vi "get desired keys.vi"(8 "error in":errorcluster, 11 "MotionModule configuration in":refnum<class "MotionModule configuration.lvclass">) -> (0 "error out":errorcluster, 2 "desired keys":string[](array[string]), 3 "MotionModule configuration out":refnum<class "MotionModule configuration.lvclass">)   [LabVIEW 2017, in "MotionModule configuration.lvclass"]
uses:
  MotionModule configuration.lvclass
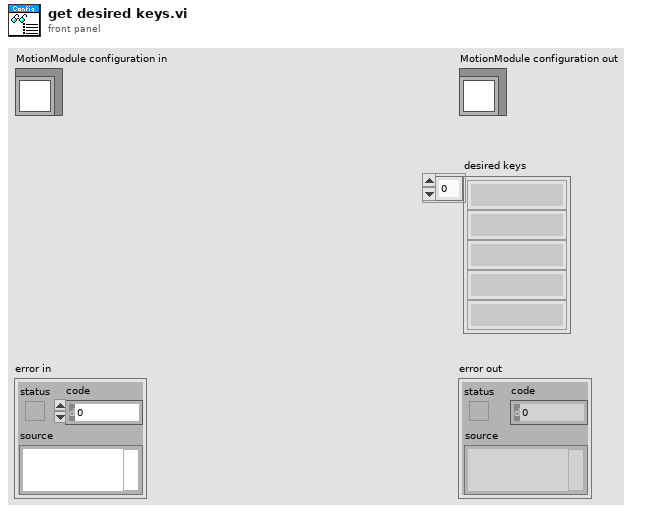
[diagram p1: front panel]
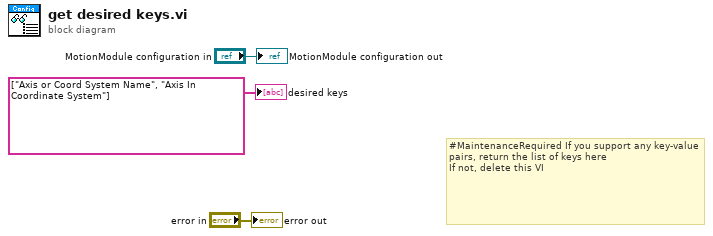
[diagram p0: block diagram]
diagram:
  # "#MaintenanceRequired If you support any key-value pairs, return the list of keys here\nIf not, delete this VI"
  "error out" <- "error in"
  "MotionModule configuration out" <- "MotionModule configuration in"
  "desired keys" <- string[] ["Axis or Coord System Name", "Axis In Coordinate System"] ("desired keys")
